vi "gRPC Status to Node Status.vi"(2 "gRPC Status":T4) -> (4 "Node Status":T1 {"Custom 8" format="%#_13g"})   [LabVIEW 2021, in "CIFTemplateCommon.lvlib"]
uses:
  CIFTemplateCommon.lvlib
  Typedef/Plugin State.ctl
  Typedef/Simple Error.ctl
  Typedef/Plugin Status.ctl
  CIFNodeCoreGrpc/CIFNodeCoreGrpc_server/RPC Messages/cif_nodecore_Error.ctl
  CIFNodeCoreGrpc/CIFNodeCoreGrpc_server/CIFNodeCoreGrpc_server.lvlib
  CIFNodeCoreGrpc/CIFNodeCoreGrpc_server/RPC Messages/cif_nodecore_StatusData_State.ctl
  CIFNodeCoreGrpc/CIFNodeCoreGrpc_server/RPC Messages/cif_nodecore_StatusData.ctl
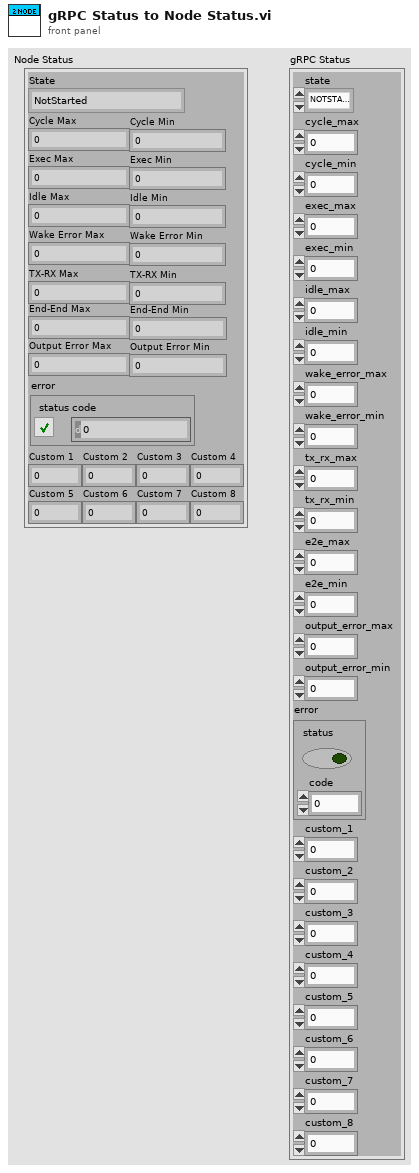
[diagram p1: front panel]
types:
  T1 = typedef "CIFTemplateCommon.lvlib/Plugin Status.ctl" = cluster{"State":T2, "Cycle Max":i32, "Cycle Min":i32, "Exec Max":i32, "Exec Min":i32, "Idle Max":i32, "Idle Min":i32, "Wake Error Max":i32, "Wake Error Min":i32, "TX-RX Max":i32, "TX-RX Min":i32, "End-End Max":i32, "End-End Min":i32, "Output Error Max":i32, "Output Error Min":i32, "error":T3, "Custom 1":u64, "Custom 2":u64, "Custom 3":u64, "Custom 4":u64, "Custom 5":dbl, "Custom 6":dbl, "Custom 7":dbl, "Custom 8":dbl}
  T2 = typedef "CIFTemplateCommon.lvlib/Plugin State.ctl" = enum32{"NotStarted", "Initialized", "Ready", "Running", "Shutdown"}
  T3 = typedef "CIFTemplateCommon.lvlib/Simple Error.ctl" = cluster{"status":bool, "code":i32}
  T4 = typedef "CIFNodeCoreGrpc_server.lvlib/cif_nodecore_StatusData.ctl" = cluster{"state":T5, "cycle_max":i32, "cycle_min":i32, "exec_max":i32, "exec_min":i32, "idle_max":i32, "idle_min":i32, "wake_error_max":i32, "wake_error_min":i32, "tx_rx_max":i32, "tx_rx_min":i32, "e2e_max":i32, "e2e_min":i32, "output_error_max":i32, "output_error_min":i32, "error":T6, "custom_1":u64, "custom_2":u64, "custom_3":u64, "custom_4":u64, "custom_5":dbl, "custom_6":dbl, "custom_7":dbl, "custom_8":dbl}
  T5 = typedef "CIFNodeCoreGrpc_server.lvlib/cif_nodecore_StatusData_State.ctl" = enum32{"NOTSTARTED", "INITIALIZED", "READY", "RUNNING", "SHUTDOWN"}
  T6 = typedef "CIFNodeCoreGrpc_server.lvlib/cif_nodecore_Error.ctl" = cluster{"status":bool, "code":i32}
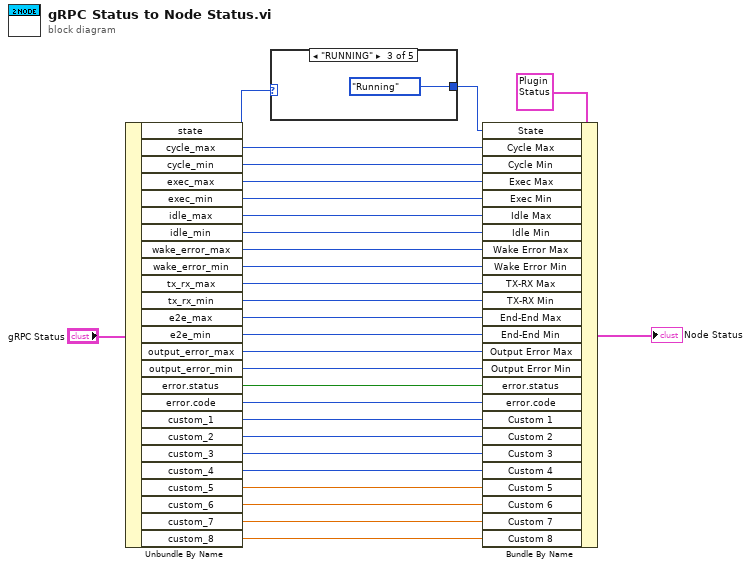
[diagram p0: block diagram]
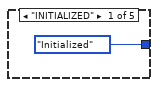
[diagram p2: hidden frame]
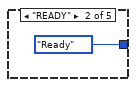
[diagram p3: hidden frame]
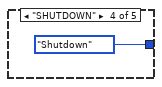
[diagram p4: hidden frame]
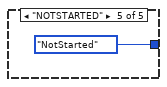
[diagram p5: hidden frame]
diagram:
  n1 = Unbundle By Name("gRPC Status") -> ("state"=w29:T5, "cycle_max"=w28:i32, "cycle_min"=w27:i32, "exec_max"=w26:i32, "exec_min"=w25:i32, "idle_max"=w24:i32, "idle_min"=w23:i32, "wake_error_max"=w22:i32, "wake_error_min"=w21:i32, "tx_rx_max"=w20:i32, "tx_rx_min"=w19:i32, "e2e_max"=w18:i32, "e2e_min"=w17:i32, "output_error_max"=w16:i32, "output_error_min"=w15:i32, "error.status"=w14:bool, "error.code"=w13:i32, "custom_1"=w5:u64, "custom_2"=w6:u64, "custom_3"=w7:u64, "custom_4"=w8:u64, "custom_5"=w9:dbl, "custom_6"=w10:dbl, "custom_7"=w11:dbl, "custom_8"=w12:dbl)
  n2 = case shown="\"RUNNING\"" w29 {
    tunnel: [Plugin_State."Initialized" ("state") Plugin_State."Ready" ("state") Plugin_State."Running" ("state") Plugin_State."Shutdown" ("state") Plugin_State."NotStarted" ("State")] -> w1
    frame "INITIALIZED" {
    }
    frame "READY" {
    }
    frame "RUNNING" {
    }
    frame "SHUTDOWN" {
    }
    frame "NOTSTARTED" {
    }
  }
  n3 = Bundle By Name(cluster=T1 {"State"=enum."NotStarted", "Cycle Max"=0, "Cycle Min"=0, "Exec Max"=0, "Exec Min"=0, "Idle Max"=0, "Idle Min"=0, "Wake Error Max"=0, "Wake Error Min"=0, "TX-RX Max"=0, "TX-RX Min"=0, "End-End Max"=0, "End-End Min"=0, "Output Error Max"=0, "Output Error Min"=0, "error"={"status"=FALSE, "code"=0}, "Custom 1"=0, "Custom 2"=0, "Custom 3"=0, "Custom 4"=0, "Custom 5"=0.0, "Custom 6"=0.0, "Custom 7"=0.0, "Custom 8"=0.0} ("Node Status"), "State"=w1, "Cycle Max"=w28, "Cycle Min"=w27, "Exec Max"=w26, "Exec Min"=w25, "Idle Max"=w24, "Idle Min"=w23, "Wake Error Max"=w22, "Wake Error Min"=w21, "TX-RX Max"=w20, "TX-RX Min"=w19, "End-End Max"=w18, "End-End Min"=w17, "Output Error Max"=w16, "Output Error Min"=w15, "error.status"=w14, "error.code"=w13, "Custom 1"=w5, "Custom 2"=w6, "Custom 3"=w7, "Custom 4"=w8, "Custom 5"=w9, "Custom 6"=w10, "Custom 7"=w11, "Custom 8"=w12) -> (→"Node Status":T1)
